vi "Destroy.vi"(8 "error in (no error)":errorcluster, 11 "I2C Bus in":refnum<class "I2C Bus.lvclass">) -> (0 "error out":errorcluster)   [LabVIEW 2020, in "I2C Bus.lvclass"]
uses:
  I2C Bus.lvclass
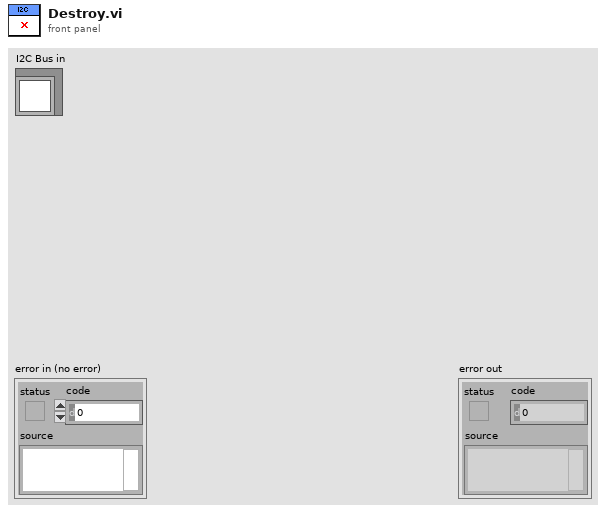
[diagram p1: front panel]
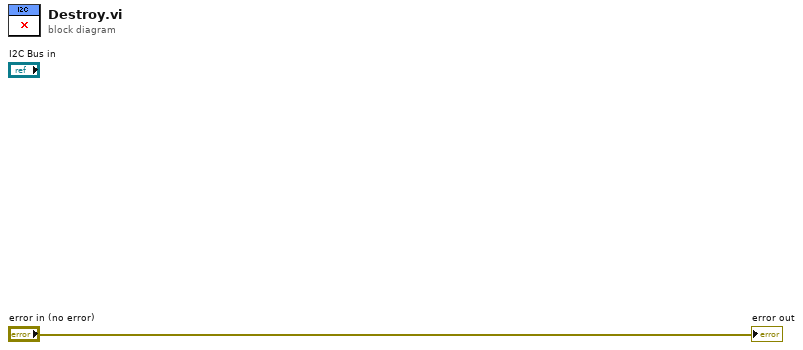
[diagram p0: block diagram]
diagram:
  "error out" <- "error in (no error)"
